vi "Get Data (All Elements).vi"(7 "Start index [0]":i32, 8 "error in (no error)":errorcluster, 10 "Data [name]":T1=enum."name", 11 "Composite Object in":refnum<class "CConfig Object.lvclass">) -> (0 "error out":errorcluster, 2 "Data":string[](array[string]), 3 "Composite Object out":refnum<class "CConfig Object.lvclass">, 4 "First part":i32)   [LabVIEW 2013, in "CConfig Object.lvclass"]
doc: "Copyright 2018, Carya Automatisering, Wiebe Walstra."
uses:
  CConfig Object.lvclass
  Data.ctl
  CConfig Object.lvclass/CConfig Object.ctl
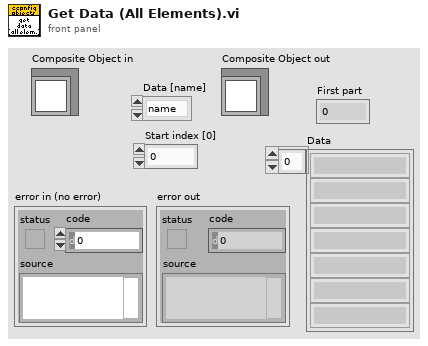
[diagram p1: front panel]
types:
  T1 = typedef "CConfig Object.lvclass/Data.ctl" = enum16{"pre", "name", "middle", "value", "post", "newline", "persistant", "tagged", "type"}
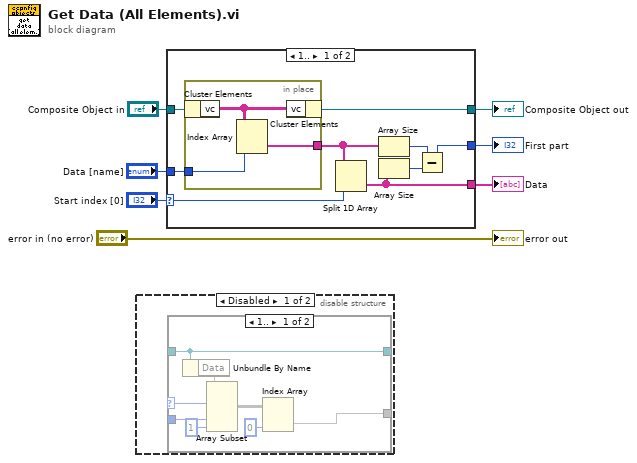
[diagram p0: block diagram]
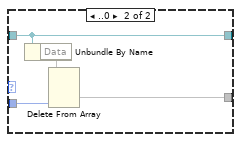
[diagram p2: hidden frame]
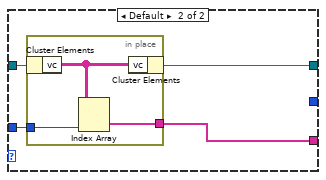
[diagram p4: hidden frame]
diagram:
  n1 = disable-structure shown="Disabled" {
    frame Disabled {
      n2 = case shown="1.." {
        selector: _ -> [w9 _]
        tunnel: [w15 w16] -> _
        tunnel: _ -> [w14 w17]
        tunnel: _ -> [w10 w19]
        tunnel: [w10 w19] -> _
        frame 1.. {
          n3 = Unbundle By Name(w10) -> ("Data"=w13)
          n4 = Array Subset(array=w13, index (row)=w9, index (col)=w14, length (col)=1 ("length")) -> (w12:void[][])  [unwired: 1 in]
          n5 = Index Array(array=w12, index (col)=0 ("disabled index (col)")) -> (element=w15:void[])  [unwired: 1 in]
        }
        frame ..0 {
          n6 = Unbundle By Name(w19) -> ("Data"=w18)
          n7 = Delete From Array(array=w18, index (col)=w17) -> (deleted portion=w16)  [unwired: 2 in, 1 out]
        }
      }
    }
    frame Enabled {
    }
  }
  n8 = case shown="1.." "Start index [0]" {
    selector: "Start index [0]" -> [w25 _]
    tunnel: [w23 w32] -> w6
    tunnel: "Data [name]" -> [w26 w33]
    tunnel: "Composite Object in" -> [w28 w35]
    tunnel: [w27 w34] -> w3
    tunnel: [w20 _] -> w1
    frame 1.. {
      n9 = in-place {
        in-place-border: [w31] -> w24
        in-place-border: w26 -> [w30]
        n10 = in-place-cluster #1(w28) -> ("vc"=w29:string[][])
        n11 = Index Array(array=w29, index (col)=w30) -> (element=w31:string[])  [unwired: 1 in]
        n12 = in-place-cluster #1("vc"=w29) -> (w27:refnum<class "CConfig Object.lvclass">)
      }
      n13 = Split 1D Array(array=w24, index=w25) -> (second subarray=w23:string[])  [unwired: 1 out]
      n14 = Array Size(array=w24) -> (size(s)=w22:i32)
      n15 = Array Size(array=w23) -> (size(s)=w21:i32)
      n16 = Subtract(x=w22, y=w21) -> (x-y=w20:i32)
    }
    frame Default {
      n17 = in-place {
        in-place-border: [w38] -> w32
        in-place-border: w33 -> [w37]
        n18 = in-place-cluster #2(w35) -> ("vc"=w36:string[][])
        n19 = Index Array(array=w36, index (col)=w37) -> (element=w38:string[])  [unwired: 1 in]
        n20 = in-place-cluster #2("vc"=w36) -> (w34:refnum<class "CConfig Object.lvclass">)
      }
    }
  }
  "Composite Object out" <- w3
  "Data" <- w6
  "First part" <- w1
  "error out" <- "error in (no error)"
